vi "上下限图表.vi"() -> ()   [LabVIEW 2012]
panel:
  in  "偏移量":dbl
  in  "上限":dbl=10.0
  in  "停止":bool
  out "波形图表":cluster{dbl, "随机数":dbl, dbl}(graph)
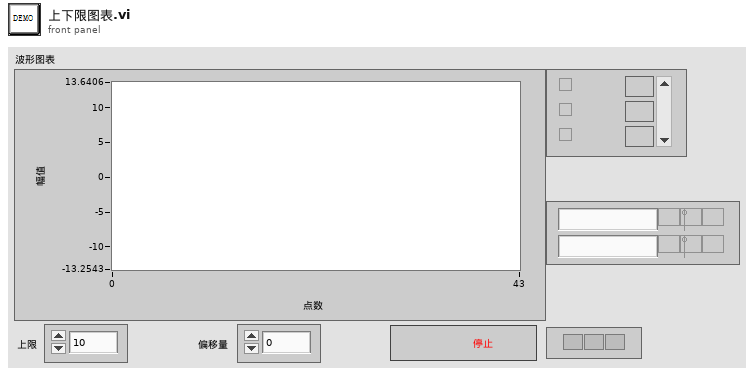
[diagram p1: front panel]
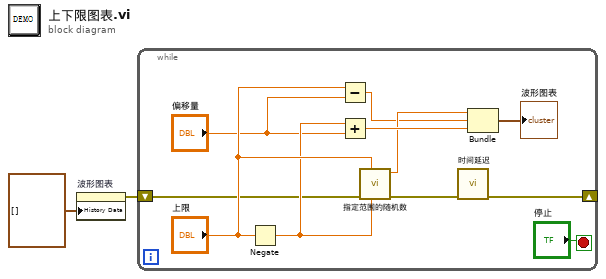
[diagram p0: block diagram]
diagram:
  n1 = property on="波形图表" class="WFChart (严格)"("History Data"=cluster{dbl, "随机数":dbl, dbl}[] [] ("历史数据")) -> (error out=w1:errorcluster)  [unwired: 2 in, 1 out]
  n2 = while {
    shift-right: [w5] -> _
    shift-left: w1 -> [w6]
    stop <- "停止" stop-if-true
    n3 = Negate(x="上限") -> (-x=w10:dbl)
    n4 = Subtract(x="上限", y="偏移量") -> (x-y=w3:dbl)
    n5 = Add(x=w10, y="偏移量") -> (x+y=w8:dbl)
    n6 = call-poly "指定范围的随机数.vi"("下限 (0.00)"=w10, "上限 (1.00)"="上限", "Error In"=w6) -> ("Error Out"=w13:errorcluster, "随机数"=w4:dbl)  [unwired: 7 in]
    n7 = call "时间延迟"("error in (no error)"=w13) -> ("error out"=w5:errorcluster)  [unwired: 10 in]
    n8 = Bundle("随机数"=w4, w3, w8) -> (→"波形图表":cluster{"随机数":dbl, dbl, dbl})  [unwired: 1 in]
  }
